vi "Get Multiple Tags Core.vi"(7 "Force Data Conversion? (F)":bool, 8 "error in (no error)":errorcluster, 10 "Cluster":variant, 11 "uData in":refnum<class "uData.lvclass">) -> (0 "error out":errorcluster, 2 "data":variant, 3 "uData out":refnum<class "uData.lvclass">, 4 "all found?":bool, 6 "found tags":string[](array[string]))   [LabVIEW 2023, in "uData.lvlib" / "uData.lvclass"]
doc: "Wire in a cluster with <B>LABELLED</B> elements. The cluster will be broken into individual elements, each element is used to read the corresponding tag. \nNested clusters use a label[dot]sublabel notation.\n\nWiring non-cluster datatypes or clusters with unlabelled element will throw out a runtime error.\n\nDo NOT use for handling data at high rates. This VI does not support inlining and has a high overhead due to data type conversion. Use only when convenience is required for generic messaging. However, the basic accessor methods are more efficient for recurring high rate VI calls"
uses:
  uData.lvclass
  uData.lvclass/uData.ctl
  Inline Read.vi
  Condition Tag Names.vi
  Condition Tag Name.vi
  Blank Key Reserved String.vi
  <vilib>/Utility/error.llb/Error Cluster From Error Code.vi
  <vilib>/Utility/Data Type/NI_Data Type.lvlib
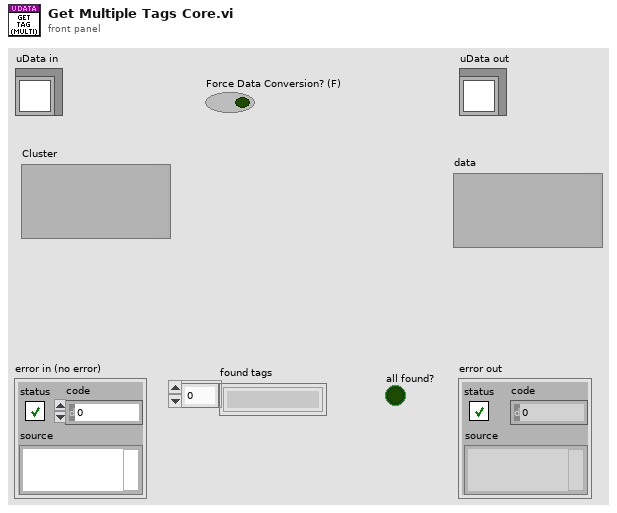
[diagram p1: front panel]
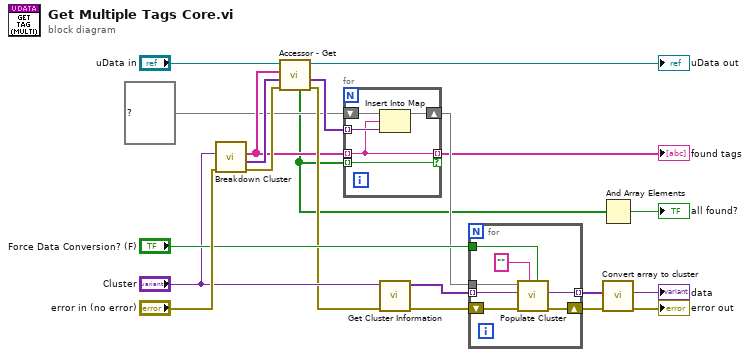
[diagram p0: block diagram]
diagram:
  n1 = call "Breakdown Cluster.vi"("error in (no error)"="error in (no error)", "Cluster"="Cluster") -> ("error out"=w8:errorcluster, "values"=w9:variant[], "tags"=w6:string[])  [unwired: 7 in]
  n2 = call "Accessor - Get.vi"("error in (no error)"=w8, "default values"=w9, "keys"=w6, "uData in"="uData in") -> ("error out"=w7:errorcluster, "values"=w5:variant[], "uData out"=→"uData out":refnum<class "uData.lvclass">, "found?"=w1:bool[])  [unwired: 4 in]
  n3 = for {
    tunnel: w6 -> [w23] mode=indexing
    tunnel: w5 -> [w26] mode=indexing
    shift-right: [w24] -> w3
    shift-left: map{string, variant} {} ("map out") -> [w25]
    tunnel: w1 -> [w22] mode=indexing
    tunnel: [w23] -> w2 mode=indexing if=w22
    n4 = Insert Into Map(map in=w25, key=w23, value=w26) -> (map out=w24:map{string, variant})  [unwired: 2 out]
  }
  "found tags" <- w2
  n5 = call <vilib>:"Get Cluster Information.vi"("error in (no error)"=w7, "variant"="Cluster") -> ("error out"=w20:errorcluster, "cluster elements"=w19:variant[])  [unwired: 8 in]
  n6 = for {
    tunnel: w19 -> [w32] mode=indexing
    tunnel: w3 -> [w31]
    shift-right: [w30] -> w16
    shift-left: w20 -> [w33]
    tunnel: [w28] -> w17 mode=indexing
    tunnel: "Force Data Conversion? (F)" -> [w27]
    n7 = call "Populate Cluster.vi"("Force Data Conversion? (F)"=w27, "prefix"="", "error in (no error)"=w33, "data in"=w32, "Map"=w31) -> ("error out"=w30:errorcluster, "data out"=w28:variant)  [unwired: 3 in, 2 out]
  }
  n8 = And Array Elements(Boolean array=w1) -> (logical AND=→"all found?":bool)
  n9 = call "Convert array to cluster.vi"("error in (no error)"=w16, "array"=w17) -> ("error out"=→"error out":errorcluster, "cluster"=→"data":variant)  [unwired: 8 in]
